vi "Netburner_cntl6.vi"(0 "Tune DAC":i32 min=0 max=3 step=1, 1 "Tune Volt":dbl=1.0 min=-9.9 max=9.9 step=0.0005 format="%_5g", 2 "NMR ADC":i32 min=0 max=3 step=1, 3 "Offset DAC":i32=1 min=0 max=3 step=1, 4 "Offset Volt":dbl=-1.0 min=-9.9 max=9.9 step=0.0005 format="%_4g", 5 "# Data":i32=100 min=1 max=500 step=1, 8 "# f steps":i32=100 min=1 max=1000 step=1) -> (6 "ADC value":dbl[](array[numeric])=[0.396, 0.3463, 0.2876, 0.2228, 0.1537, 0.0805, 0.0045, -0.0702, -0.1431, -0.2137, -0.2794, -0.3385, -0.39, -0.4334, -0.466, -0.4873, -0.4978, -0.4975, -0.4844, -0.46, -0.4257, -0.3819, -0.328, -0.2665, -0.2001, -0.1283, -0.053, 0.0228, 0.0971, 0.1707, 0.2402, 0.3035, 0.3595, 0.4081, 0.4472, 0.4748, 0.4917, 0.4981, 0.4922, 0.474, 0.4457, 0.4074, 0.359, 0.3016, 0.2385, 0.1695, 0.0959, 0.0204, -0.055, -0.1293, -0.2018, -0.2684, -0.3288, -0.3822, -0.4271, -0.4609, -0.4842, -0.4972, -0.4985, -0.4871, -0.4647, -0.4326, -0.3896, -0.337, -0.2772, -0.2116, -0.1399, -0.065, 0.0105, 0.0855, 0.1596, 0.2299, 0.2937, 0.3515, 0.4014, 0.4417, 0.4708, 0.4902, 0.4981, 0.4936, 0.4776, 0.4514, 0.4145, 0.3671, 0.3116, 0.2495, 0.181, 0.1075, 0.0328, -0.0429, -0.1179, -0.1908, -0.258, -0.3197, -0.3748, -0.4207, -0.456, -0.4814, -0.4964, -0.4988], 7 "ADC error":dbl[](array[numeric])=[0.011, 0.012, 0.0135, 0.0155, 0.0168, 0.0162, 0.0168, 0.0175, 0.0163, 0.0149, 0.0142, 0.0133, 0.0102, 0.0081, 0.0066, 0.0042, 0.0008, 0.0018, 0.0035, 0.0067, 0.0095, 0.0111, 0.0122, 0.0148, 0.0161, 0.0164, 0.0165, 0.0175, 0.017, 0.0155, 0.0148, 0.0141, 0.0119, 0.009, 0.0079, 0.0055, 0.0024, 0.001, 0.0021, 0.0049, 0.0082, 0.01, 0.0112, 0.0134, 0.0158, 0.0159, 0.0163, 0.0173, 0.0176, 0.016, 0.0153, 0.0149, 0.0132, 0.0104, 0.0087, 0.0074, 0.0039, 0.0012, 0.0014, 0.0031, 0.0067, 0.009, 0.0103, 0.0123, 0.0148, 0.0158, 0.0158, 0.0171, 0.0175, 0.0169, 0.0155, 0.0156, 0.0142, 0.0118, 0.0097, 0.0086, 0.0058, 0.0023, 0.001, 0.0018, 0.0047, 0.008, 0.0091, 0.0111, 0.0137, 0.0153, 0.0154, 0.0163, 0.0177, 0.0171, 0.0161, 0.0156, 0.0155, 0.0128, 0.0109, 0.0095, 0.0076, 0.004, 0.0016, 0.0009], 9 "Max ADC":dbl=0.4981 format="%#_5g", 10 "Min ADC":dbl=-0.4988 format="%#_5g")   [LabVIEW 2013]
uses:
  <vilib>/Analysis/NI_AALBase.lvlib
panel:
  out "ADC Voltage Chart":dbl(graph)=-0.4988
  out "# Cycles":i32=100
  out "ADC Std Dev":dbl=0.011067 format="%#_4g"
  out "Mean ADC":dbl=-0.022115000000000006 format="%#_5g"
  out "#  Bytes Read End":u32=3
  out "End string":string="?\r\n"
  out "ADC result string":string="0 1 1 -1 0 100 100\r0 0.3960  0.0110  \r\n1 0.3463  0.0120  \r\n2 0.2876  0.0135  \r\n3 0.2228  0.0155  \r\n4 0.1537  0.0168  \r\n5 0.0805  0.0162  \r\n6 0.0045  0.0168  \r\n7 -0.0702 0.0175  \r\n8 -0.1431 0.0163  \r\n9 -0.2137 0.0149  \r\n10 -0.2794 0.0142  \r\n11 -0.3385 0.0133  \r\n12 -0.3900 0.0102  \r\n13 -0.4334 0.0081  \r\n14 -0.4660 0.0066  \r\n15 -0.4873 0.0042  \r\n16 -0.4978 0.0008  \r\n17 -0.4975 0.0018  \r\n18 -0.4844 0.0035  \r\n19 -0.4600 0.0067  \r\n20 -0.4257 0.0095  \r\n21 -0.3819 0.0111  \r\n22 -0.3280 0.0122  \r\n23 -0.2665 0.0148  \r\n24 -0.2001 0.0161  \r\n25 -0.1283 0.0164  \r\n26 -0.0530 0.0165  \r\n27 0.0228  0.0175  \r\n28 0.0971  0.0170  \r\n29 0.1707  0.0155  \r\n30 0.2402  0.0148  \r\n31 0.3035  0.0141  \r\n32 0.3595  0.0119  \r\n33 0.4081  0.0090  \r\n34 0.4472  0.0079  \r\n35 0.4748  0.0055  \r\n36 0.4917  0.0024  \r\n37 0.4981  0.0010  \r\n38 0.4922  0.0021  \r\n39 0.4740  0.0049  \r\n40 0.4457  0.0082  \r\n41 0.4074  0.0100  \r\n42 0.3590  0.0112  \r\n43 0.3016  0.0134  \r\n44 0.2385  0.0158  \r\n45 0.1695  0.0159  \r\n46 0.0959  0.0163  \r\n47 0.0204  0.0173  \r\n48 -0.0550 0.0176  \r\n49 -0.1293 0.0160  \r\n50 -0.2018 0.0153  \r\n51 -0.2684 0.0149  \r\n52 -0.3288 0.0132  \r\n53 -0.3822 0.0104  \r\n54 -0.4271 0.0087  \r\n55 -0.4609 0.0074  \r\n56 -0.4842 0.0039  \r\n57 -0.4972 0.0012  \r\n58 -0.4985 0.0014  \r\n59 -0.4871 0.0031  \r\n60 -0.4647 0.0067  \r\n61 -0.4326 0.0090  \r\n62 -0.3896 0.0103  \r\n63 -0.3370 0.0123  \r\n64 -0.2772 0.0148  \r\n65 -0.2116 0.0158  \r\n66 -0.1399 0.0158  \r\n67 -0.0650 0.0171  \r\n68 0.0105  0.0175  \r\n69 0.0855  0.0169  \r\n70 0.1596  0.0155  \r\n71 0.2299  0.0156  \r\n72 0.2937  0.0142  \r\n73 0.3515  0.0118  \r\n74 0.4014  0.0097  \r\n75 0.4417  0.0086  \r\n76 0.4708  0.0058  \r\n77 0.4902  0.0023  \r\n78 0.4981  0.0010  \r\n79 0.4936  0.0018  \r\n80 0.4776  0.0047  \r\n81 0.4514  0.0080  \r\n82 0.4145  0.0091  \r\n83 0.3671  0.0111  \r\n84 0.3116  0.0137  \r\n85 0.2495  0.0153  \r\n86 0.1810  0.0154  \r\n87 0.1075  0.0163  \r\n88 0.0328  0.0177  \r\n89 -0.0429 0.0171  \r\n90 -0.1179 0.0161  \r\n91 -0.1908 0.0156  \r\n92 -0.2580 0.0155  \r\n93 -0.3197 0.0128  \r\n94 -0.3748 0.0109  \r\n95 -0.4207 0.0095  \r\n96 -0.4560 0.0076  \r\n97 -0.4814 0.0040  \r\n98 -0.4964 0.0016  \r\n99 -0.4988 0.0009  \r\n"
  out "#  Bytes Read Data":u32=2109
  out "DAC, ADC String":string
  out "Error Out":errorcluster={"status"=FALSE, "code"=1073676294, "source"="VISA Read in Netburner_RD.vi->Netburner_cntl6.vi"}
  in  "Error In (none)":errorcluster
  in  "COM Port #":refnum<visa-resource-name>="COM3"
  # "Netburner ADC/DAC Test Interface"
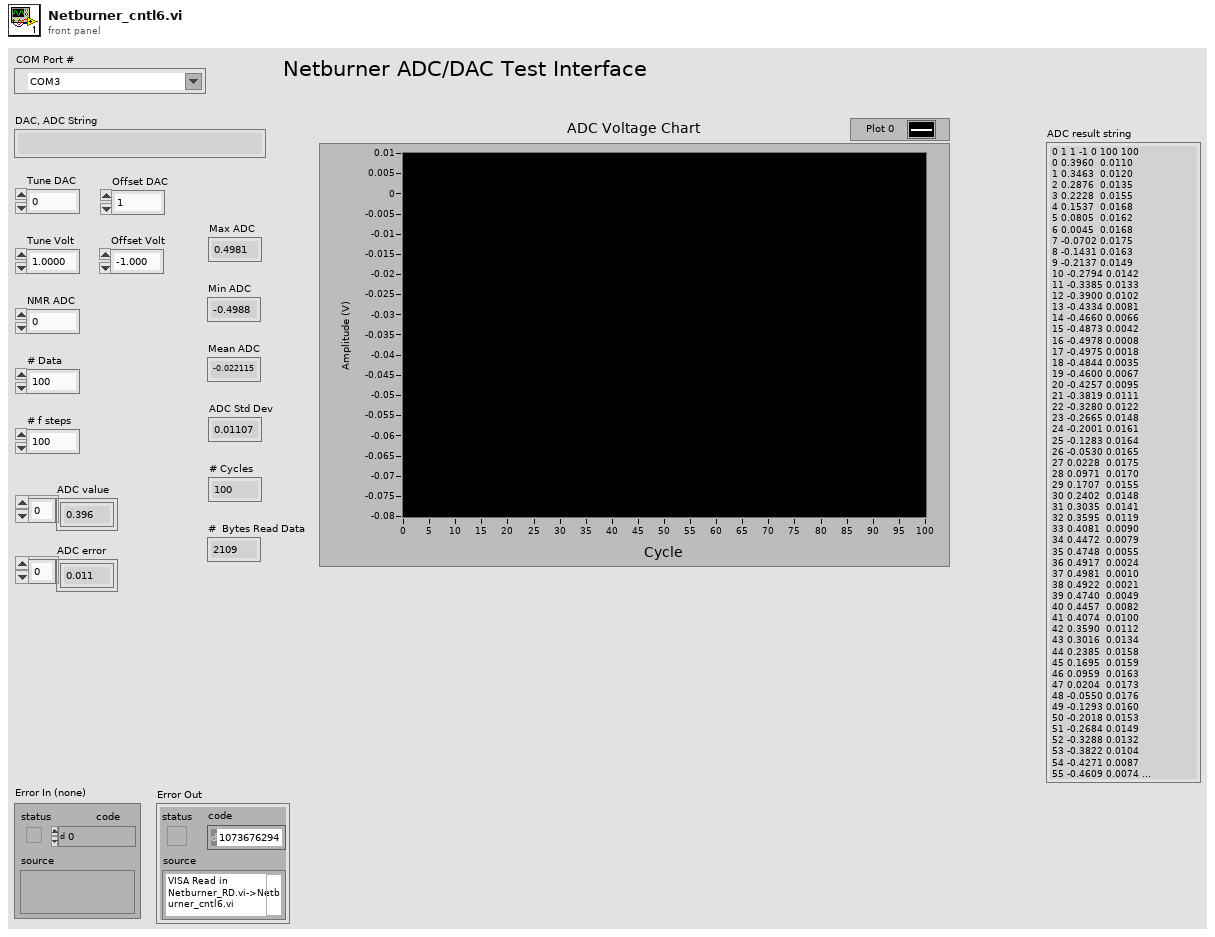
[diagram p1: front panel]
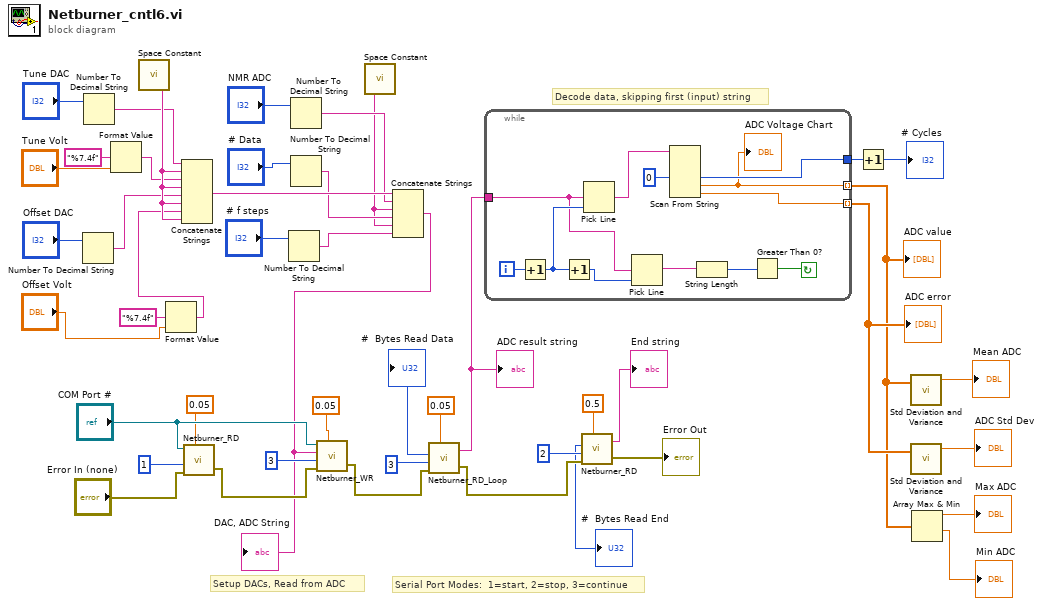
[diagram p0: block diagram]
diagram:
  # "Decode data, skipping first (input) string"
  # "Serial Port Modes:  1=start, 2=stop, 3=continue"
  # "Setup DACs, Read from ADC"
  n1 = Number To Decimal String(number="Offset DAC") -> (decimal integer string=w11:string)  [unwired: 1 in]
  n2 = Number To Decimal String(number="Tune DAC") -> (decimal integer string=w12:string)  [unwired: 1 in]
  n3 = Format Value(format string="%7.4f", value (0)="Tune Volt") -> (output string=w1:string)  [unwired: 1 in]
  n4 = call <vilib>:"Space Constant.vi"() -> ("String"=w13:string)
  n5 = Format Value(format string="%7.4f", value (0)="Offset Volt") -> (output string=w4:string)  [unwired: 1 in]
  n6 = Concatenate Strings(w12, w13, w1, w13, w11, w13, w4, w13) -> (w15:string)
  n7 = call "Netburner_RD.vi"("VISA resource name (COM Port #)"="COM Port #", "Mode (0)"=1, "Error In (no error)"="Error In (none)", "Wait (sec)"=0.05) -> ("Error Out"=w45:errorcluster)  [unwired: 2 out]
  n8 = Number To Decimal String(number="# f steps") -> (decimal integer string=w8:string)  [unwired: 1 in]
  n9 = Number To Decimal String(number="NMR ADC") -> (decimal integer string=w10:string)  [unwired: 1 in]
  n10 = Number To Decimal String(number="# Data") -> (decimal integer string=w9:string)  [unwired: 1 in]
  n11 = call <vilib>:"Space Constant.vi"() -> ("String"=w7:string)
  n12 = Concatenate Strings(w15, w10, w7, w9, w7, w8) -> (w14:string)
  "DAC, ADC String" <- w14
  n13 = call "Netburner_WR.vi"("VISA resource name (COM Port #)"="COM Port #", "String to Send"=w14, "Mode (0)"=3, "Error In (no error)"=w45, "Wait (sec)"=0.05) -> ("Error Out"=w33:errorcluster)  [unwired: 1 in]
  n14 = call "Netburner_RD_Loop.vi"("Mode (0)"=3, "Error In (no error)"=w33, "Wait (sec)"=0.05) -> ("#  Bytes Read"=→"#  Bytes Read Data":u32, "Return String from Device"=w29:string, "Error Out"=w41:errorcluster)  [unwired: 1 in]
  "ADC result string" <- w29
  n15 = while {
    tunnel: w29 -> [w49]
    tunnel: [w53] -> w25
    tunnel: [w47] -> w23 mode=indexing
    tunnel: [w52] -> w28 mode=indexing
    i -> [w58]
    stop <- w54 continue-if-true
    n16 = Increment(x=w58) -> (x+1=w51:i32)
    n17 = Increment(x=w51) -> (x+1=w50:i32)
    n18 = Pick Line(multi-line string=w49, line index=w51) -> (output string=w56:string)  [unwired: 1 in]
    n19 = Pick Line(multi-line string=w49, line index=w50) -> (output string=w48:string)  [unwired: 1 in]
    n20 = Scan From String "Scan From String"(input string=w56, default 1=0) -> (output 1=w53:i32, output 2=w47:dbl, output 3=w52:dbl)  [unwired: 5 in, 3 out]
    "ADC Voltage Chart" <- w47
    n21 = String Length(string=w48) -> (length=w55:i32)
    n22 = Greater Than 0?(x=w55) -> (x > 0?=w54:bool)
  }
  "ADC value" <- w23
  "ADC error" <- w28
  n23 = call "Netburner_RD.vi"("Mode (0)"=2, "Error In (no error)"=w41, "Wait (sec)"=0.5) -> ("Number of Bytes Received"=→"#  Bytes Read End":u32, "Return String from Device"=→"End string":string, "Error Out"=→"Error Out":errorcluster)  [unwired: 1 in]
  n24 = Increment(x=w25) -> (x+1=→"# Cycles":i32)
  n25 = call <vilib>:"Std Deviation and Variance.vi"("X"=w23) -> ("mean"=→"Mean ADC":dbl)  [unwired: 1 in, 2 out]
  n26 = call <vilib>:"Std Deviation and Variance.vi"("X"=w28) -> ("mean"=→"ADC Std Dev":dbl)  [unwired: 1 in, 2 out]
  n27 = Array Max & Min(array=w23) -> (max value=→"Max ADC":dbl, min value=→"Min ADC":dbl)  [unwired: 2 out]
